vi "Save Editor Data.vi"(8 "error in":errorcluster, 11 "TSC Button Editor":refnum<class "TSC Button Editor.lvclass">) -> (0 "error out":errorcluster)   [LabVIEW 2021, in "TSC Button Editor.lvclass"]
doc: "This VI is called when the button editor finishes to write the object-data to an XML file for loading on next launch.\n\n<b>Code Developed By:</b> +\nDaniel Coons +\nTechnology Service Corporation +\nwww.tsc.com/atcs"
uses:
  TSC Button Editor.lvclass
  TSC Button Editor.lvclass/TSC Button Editor.ctl
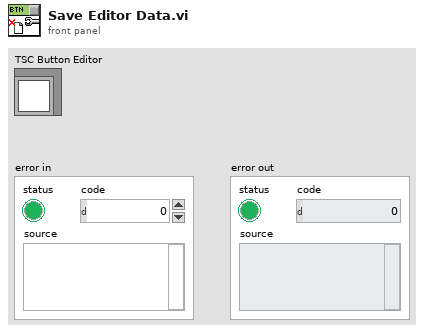
[diagram p1: front panel]
types:
  T1 = enum16{"open", "replace", "create", "open or create", "replace or create", "replace or create with confirmation"}
  T2 = cluster{"2D Picture":picture, "path":path, "image-name":string}[]
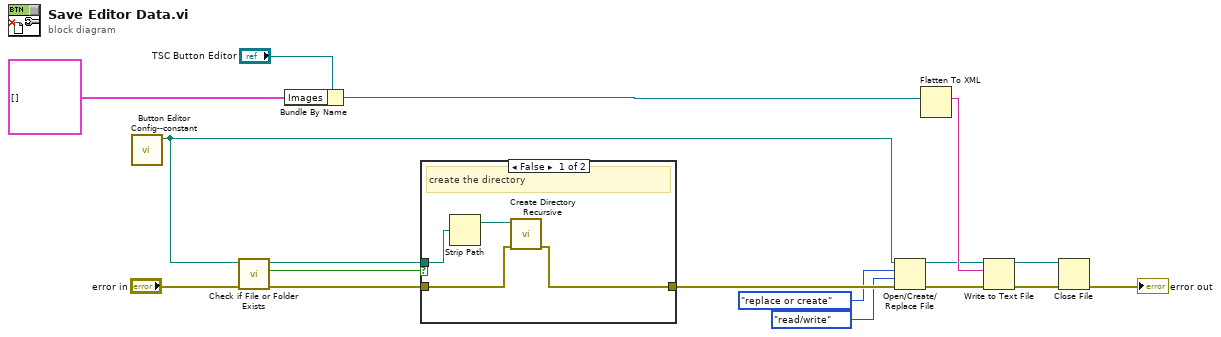
[diagram p0: block diagram]
diagram:
  n1 = call "Button Editor Config--constant.vi"() -> ("Button Editor Config"=w1:path)  [unwired: 11 in]
  n2 = call <vilib>:"Check if File or Folder Exists.vi"("error in (no error)"="error in", "path"=w1) -> ("error out"=w16:errorcluster, "file or folder exists?"=w15:bool, "dup path"=w14:path)  [unwired: 7 in]
  n3 = Bundle By Name(cluster="TSC Button Editor", "Images"=T2 []) -> (w2:refnum<class "TSC Button Editor.lvclass">)
  n4 = case shown="False" w15 {
    tunnel: w16 -> [w21 w22]
    tunnel: w14 -> [w19 _]
    tunnel: [w18 w22] -> w6
    frame False {
      # "create the directory"
      n5 = Strip Path(path=w19) -> (stripped path=w20:path)  [unwired: 1 out]
      n6 = call <vilib>:"Create Directory Recursive.vi"("error in (no error)"=w21, "directory"=w20) -> ("error out"=w18:errorcluster)  [unwired: 3 in, 2 out]
    }
    frame True {
      # "it is there, so we don't need to make dir"
    }
  }
  n7 = Open/Create/Replace File(file path (use dialog)=w1, error in=w6, operation (0:open)=T1."replace or create", access (0:read/write)=enum16{"read/write", "read-only", "write-only"}."read/write") -> (refnum out=w9:refnum<file>, error out=w7:errorcluster)  [unwired: 2 in, 1 out]
  n8 = Flatten To XML(6:w2) -> (2:w11:string)
  n9 = Write to Text File(file (use dialog)=w9, text=w11, error in=w7) -> (refnum out=w10:refnum<file>, error out=w8:errorcluster)  [unwired: 1 in, 1 out]
  n10 = Close File(refnum=w10, error in=w8) -> (error out=→"error out":errorcluster)  [unwired: 1 out]
